vi "XY Graph Get-Set Plot Style.vi"(6 "Get (F)/Set":bool, 8 "Error In":errorcluster, 9 "Plot Index":i32 caption="Plot Index (0)", 10 "Plot Style in":T1, 11 "XYGraph in":refnum<vi>) -> (0 "Error Out":errorcluster, 1 "Plot Name":string, 2 "Plot Style out":T1, 3 "Graph Caption":string)   [LabVIEW 2019]
uses:
  XY Graph Plot Properties.ctl
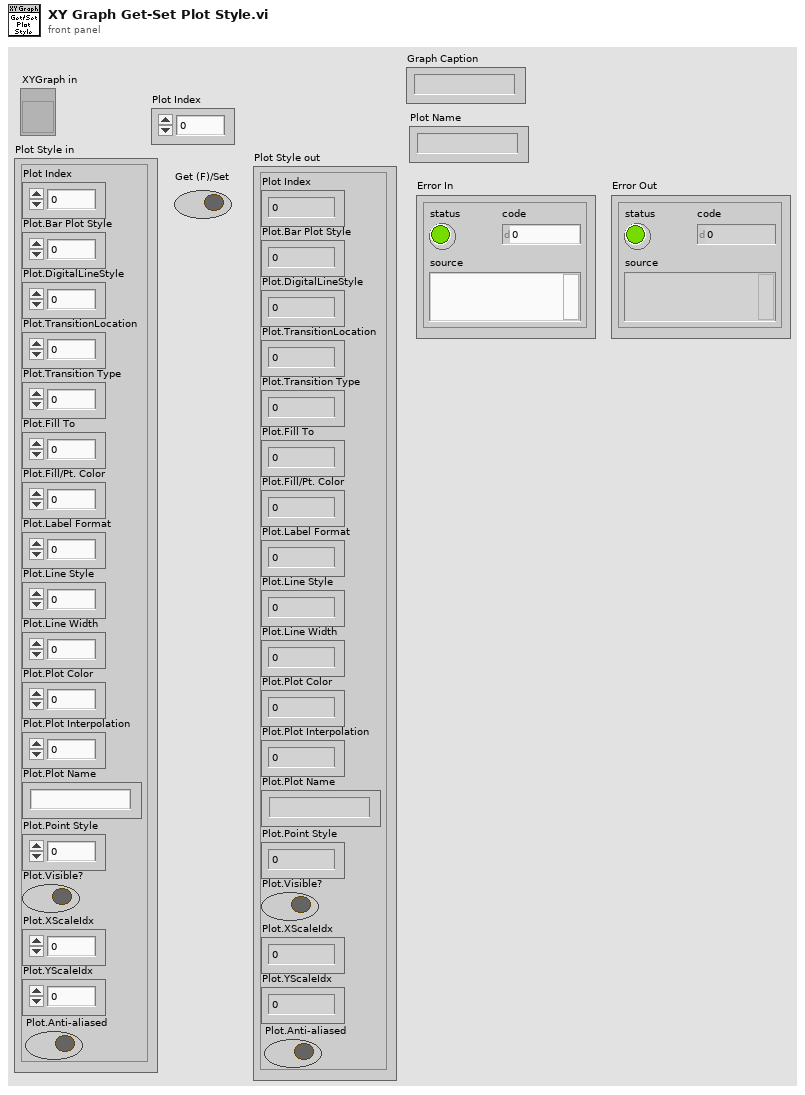
[diagram p1: front panel]
types:
  T1 = typedef "XY Graph Plot Properties.ctl" = cluster{"Plot Index":i32, "Plot.Bar Plot Style":u8, "Plot.DigitalLineStyle":u8, "Plot.TransitionLocation":u8, "Plot.Transition Type":u8, "Plot.Fill To":i16, "Plot.Fill/Pt. Color":u32, "Plot.Label Format":u8, "Plot.Line Style":u8, "Plot.Line Width":u8, "Plot.Plot Color":u32, "Plot.Plot Interpolation":u8, "Plot.Plot Name":string, "Plot.Point Style":u8, "Plot.Visible?":bool, "Plot.XScaleIdx":u32, "Plot.YScaleIdx":u32, "Plot.Anti-aliased":bool}
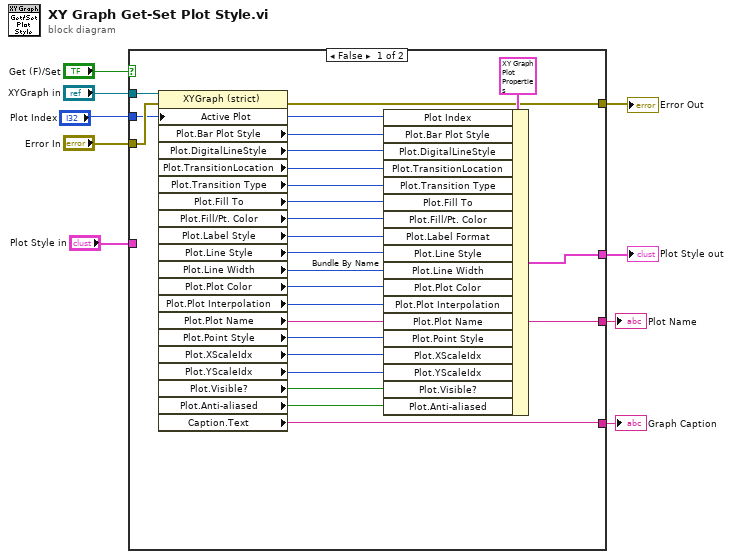
[diagram p0: block diagram]
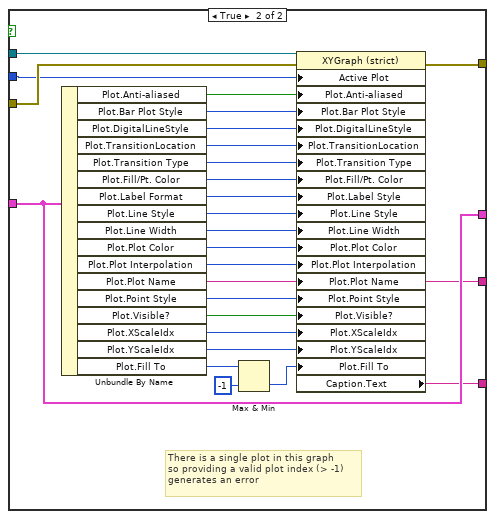
[diagram p2: hidden frame]
diagram:
  n1 = case shown="False" "Get (F)/Set" {
    tunnel: "XYGraph in" -> [w33 w58]
    tunnel: "Plot Index" -> [w30 w56]
    tunnel: "Error In" -> [w32 w57]
    tunnel: [w14 w54] -> w5
    tunnel: [w13 w55] -> w4
    tunnel: "Plot Style in" -> [_ w54]
    tunnel: [w11 w35] -> w2
    tunnel: [w10 w34] -> w1
    frame False {
      n2 = property class="XYGraph (strict)"(reference=w33, error in=w32, "Active Plot"=w30) -> (error out=w13:errorcluster, "Plot.Bar Plot Style"=w29:u8, "Plot.DigitalLineStyle"=w28:u8, "Plot.TransitionLocation"=w27:u8, "Plot.Transition Type"=w25:u8, "Plot.Fill To"=w26:i16, "Plot.Fill/Pt. Color"=w24:u32, "Plot.Label Style"=w23:u8, "Plot.Line Style"=w22:u8, "Plot.Line Width"=w21:u8, "Plot.Plot Color"=w20:u32, "Plot.Plot Interpolation"=w19:u8, "Plot.Plot Name"=w11:string, "Plot.Point Style"=w18:u8, "Plot.XScaleIdx"=w17:u32, "Plot.YScaleIdx"=w16:u32, "Plot.Visible?"=w15:bool, "Plot.Anti-aliased"=w12:bool, "Caption.Text"=w10:string)  [unwired: 1 out]
      n3 = Bundle By Name(cluster=T1 {"Plot Index"=0, "Plot.Bar Plot Style"=0, "Plot.DigitalLineStyle"=0, "Plot.TransitionLocation"=0, "Plot.Transition Type"=0, "Plot.Fill To"=0, "Plot.Fill/Pt. Color"=0, "Plot.Label Format"=0, "Plot.Line Style"=0, "Plot.Line Width"=0, "Plot.Plot Color"=0, "Plot.Plot Interpolation"=0, "Plot.Plot Name"="", "Plot.Point Style"=0, "Plot.Visible?"=FALSE, "Plot.XScaleIdx"=0, "Plot.YScaleIdx"=0, "Plot.Anti-aliased"=FALSE} ("input cluster"), "Plot Index"=w30, "Plot.Bar Plot Style"=w29, "Plot.DigitalLineStyle"=w28, "Plot.TransitionLocation"=w27, "Plot.Transition Type"=w25, "Plot.Fill To"=w26, "Plot.Fill/Pt. Color"=w24, "Plot.Label Format"=w23, "Plot.Line Style"=w22, "Plot.Line Width"=w21, "Plot.Plot Color"=w20, "Plot.Plot Interpolation"=w19, "Plot.Plot Name"=w11, "Plot.Point Style"=w18, "Plot.XScaleIdx"=w17, "Plot.YScaleIdx"=w16, "Plot.Visible?"=w15, "Plot.Anti-aliased"=w12) -> (w14:T1)
    }
    frame True {
      # "There is a single plot in this graph\nso providing a valid plot index (> -1)\ngenerates an error"
      n4 = Unbundle By Name(w54) -> ("Plot.Anti-aliased"=w53:bool, "Plot.Bar Plot Style"=w52:u8, "Plot.DigitalLineStyle"=w51:u8, "Plot.TransitionLocation"=w50:u8, "Plot.Transition Type"=w49:u8, "Plot.Fill/Pt. Color"=w48:u32, "Plot.Label Format"=w44:u8, "Plot.Line Style"=w43:u8, "Plot.Line Width"=w42:u8, "Plot.Plot Color"=w41:u32, "Plot.Plot Interpolation"=w40:u8, "Plot.Plot Name"=w35:string, "Plot.Point Style"=w39:u8, "Plot.Visible?"=w38:bool, "Plot.XScaleIdx"=w37:u32, "Plot.YScaleIdx"=w36:u32, "Plot.Fill To"=w46:i16)
      n5 = Max & Min(x=w46, y=i16 -1 ("Plot.Fill To")) -> (min(x,y)=w45:i16)  [unwired: 1 out]
      n6 = property class="XYGraph (strict)"(reference=w58, error in=w57, "Active Plot"=w56, "Plot.Anti-aliased"=w53, "Plot.Bar Plot Style"=w52, "Plot.DigitalLineStyle"=w51, "Plot.TransitionLocation"=w50, "Plot.Transition Type"=w49, "Plot.Fill/Pt. Color"=w48, "Plot.Label Style"=w44, "Plot.Line Style"=w43, "Plot.Line Width"=w42, "Plot.Plot Color"=w41, "Plot.Plot Interpolation"=w40, "Plot.Plot Name"=w35, "Plot.Point Style"=w39, "Plot.Visible?"=w38, "Plot.XScaleIdx"=w37, "Plot.YScaleIdx"=w36, "Plot.Fill To"=w45) -> (error out=w55:errorcluster, "Caption.Text"=w34:string)  [unwired: 1 out]
    }
  }
  "Plot Style out" <- w5
  "Error Out" <- w4
  "Plot Name" <- w2
  "Graph Caption" <- w1
